vi "Stoerungen (257-320) - Amium.vi"(8 "Fehler (Eingang)":errorcluster caption="Fehler (Eingang, kein Fehler)") -> (0 "Fehler (Ausgang)":errorcluster, 3 "Störungen 257-320":u64)   [LabVIEW 2020, in "Stoerungen.lvlib"]
uses:
  Stoerungen.lvlib
  Seiten/System Einstellungen V2/Aktioen FGV System.ctl
  cRIO/Stoermeldungen/Stoerungen 257-320.ctl
  Stoerungen Messgeraet/Aktionen Kommunikation Stoerung.ctl
  Amium PNS/Aktion FGV Amium Daten.ctl
  PNS/Parameternamen PNS.ctl
  PNS/PNS.lvlib
  Seiten/System Einstellungen V2/System Einstellungen V2.lvlib
  cRIO/Stoermeldungen/Stoermeldungen.lvlib
  Amium PNS/Amium PNS.lvlib
panel:
  # "Störmeldungen PNS (257-320)"
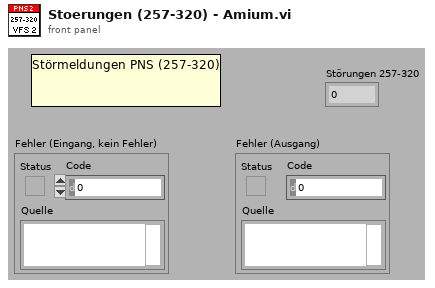
[diagram p1: front panel]
types:
  T1 = typedef "System Einstellungen V2.lvlib/Aktioen FGV System.ctl" = enum16{"lesen", "laden", "speichern", "Optionen schreiben", "Zeitstempel", "Reset BMP", "Reset SQP", "Wartung", "Werkseinstellung"}
  T2 = typedef "System Einstellungen V2.lvlib/Optionen.ctl" = cluster{"Störmeldep.":bool, "Betriebszustände":bool, "AK in ppm":bool, "log Cal-Gas":bool, "log 0-Gas":bool, "Durchflusssensor 0-5V":bool, "PNS?":bool, "Mit N2 spülen":bool, "TRE08":bool, "Amium 10-Fach":bool, "Verticale Scrollbar aktiv":bool, "Loggingtakt":bool, "AK Rezeptwechsel gleich wie MKS":bool, "NG ECO":bool}
  T3 = typedef "Amium PNS.lvlib/Aktion FGV Amium Daten.ctl" = enum16{"lesen", "Komm Daten", "Daten", "Error", "Regler", "Grenzwerte", "laden", "speichern"}
  T4 = typedef "Stoerungen.lvlib/Aktionen Kommunikation Stoerung.ctl" = enum16{"lesen", "init", "FT-IR Komm", "FT-IR Betriebsart", "FT-IR Hintergrund", "cRIO Komm", "PNS Komm", "Dichtheitstest", "Life Bit", "FTIR Komm AK", "PMA Komm", "FID Komm", "PMA Cal", "FID Ch4 Cal", "FID THC Cal", "Cal Timeout", "VFS 1 Komm", "VFS 2 Komm", "VFS 3 Komm", "VFS 4 Komm", "TRE 08 Komm", "CG-Test vorzeitig", "CG-Test Span 1", "CG-Test Span 2", "CG-Test Span 3", "CG-Test Messgas", "CG-Test löschen", "Test", "Amium AK", "AK Recept konfig", "AK Name konfig", "AK EKFG konfig"}
  T5 = typedef "Stoermeldungen.lvlib/Stoerungen 257-320.ctl" = cluster{"ERR. 257":bool, "ERR. 258":bool, "ERR. 259":bool, "ERR. 260":bool, "ERR. 261":bool, "ERR. 262":bool, "ERR. 263":bool, "ERR. 264":bool, "ERR. 265":bool, "ERR. 266":bool, "ERR. 267":bool, "ERR. 268":bool, "ERR. 269":bool, "ERR. 270":bool, "ERR. 271":bool, "ERR. 272":bool, "ERR. 273":bool, "ERR. 274":bool, "ERR. 275":bool, "ERR. 276":bool, "ERR. 277":bool, "ERR. 278":bool, "ERR. 279":bool, "ERR. 280":bool, "ERR. 281":bool, "ERR. 282":bool, "ERR. 283":bool, "ERR. 284":bool, "ERR. 285":bool, "ERR. 286":bool, "ERR. 287":bool, "ERR. 288":bool, "ERR. 289":bool, "ERR. 290":bool, "ERR. 291":bool, "ERR. 292":bool, "ERR. 293":bool, "ERR. 294":bool, "ERR. 295":bool, "ERR. 296":bool, "ERR. 297":bool, "ERR. 298":bool, "ERR. 299":bool, "ERR. 300":bool, "ERR. 301":bool, "ERR. 302":bool, "ERR. 303":bool, "ERR. 304":bool, "ERR. 305":bool, "ERR. 306":bool, "ERR. 307":bool, "ERR. 308":bool, "ERR. 309":bool, "ERR. 310":bool, "ERR. 311":bool, "ERR. 312":bool, "ERR. 313":bool, "ERR. 314":bool, "ERR. 315":bool, "ERR. 316":bool, "ERR. 317":bool, "ERR. 318":bool, "ERR. 319":bool, "ERR. 320":bool}
  T6 = typedef "PNS.lvlib/Parameternamen PNS.ctl" = enum16{"Heizkreis 1", "Heizkreis 2", "Heizkreis 3", "Heizkreis 4", "Heizkreis 5", "Heizkreis 6", "Heizkreis 7", "Heizkreis 8"}
  T7 = typedef "Amium PNS.lvlib/Amium ErrorCluster.ctl" = cluster{"Messgasdruck":bool, "Temperatur":bool, "Steuerluft":bool, "Temperatur HL 1":bool, "Temperatur HL 2":bool, "Temperatur HL 3":bool, "Temperatur HL 4":bool, "Temperatur HL 5":bool, "Temperatur HL 6":bool, "Temperatur HL 7":bool, "Temperatur HL 8":bool, "Temperatur HL 9":bool, "Temperatur HL 10":bool, "Temperatur 11 Ofen MGF/Filter":bool, "Temperatur HL12":bool, "Temperatur 13 Ofen MGP/Pumpe":bool, "Temperatur HL 14":bool}
  T8 = typedef "Amium PNS.lvlib/Temperaturregler Cluster.ctl" = cluster{"Istwert":sgl, "Sollwert":sgl, "Stellgröße":sgl, "Status":sgl, "Error":sgl}
  T9 = typedef "Stoerungen.lvlib/Stoerungen Messgeraete.ctl" = cluster{"FT-IR Komm":bool, "FT-IR Betriebsart":bool, "FT-IR Hintergrundscan":bool, "Dichtheitstest":bool, "cRIO Komm":bool, "PNS Komm":bool, "Life Bit":bool, "FT-IR AK Komm":bool, "PMA Komm":bool, "FID Komm":bool, "PMA Cal":bool, "FID CH4 Cal":bool, "FID THC Cal":bool, "Cal Timeout":bool, "VFS 1 Komm":bool, "VFS 2 Komm":bool, "VFS 3 Komm":bool, "VFS 4 Komm":bool, "TRE 08 Komm":bool, "CG-Test":bool, "CG-Test 1":bool, "CG-Test 2":bool, "CG-Test 3":bool, "Messgas - Eingang":bool, "Amium AK Komm":bool, "AK Rezept nicht konfiguriert ":bool, "AK Name nicht konfiguriert":bool, "AK EKFG nicht konfiguriert":bool}
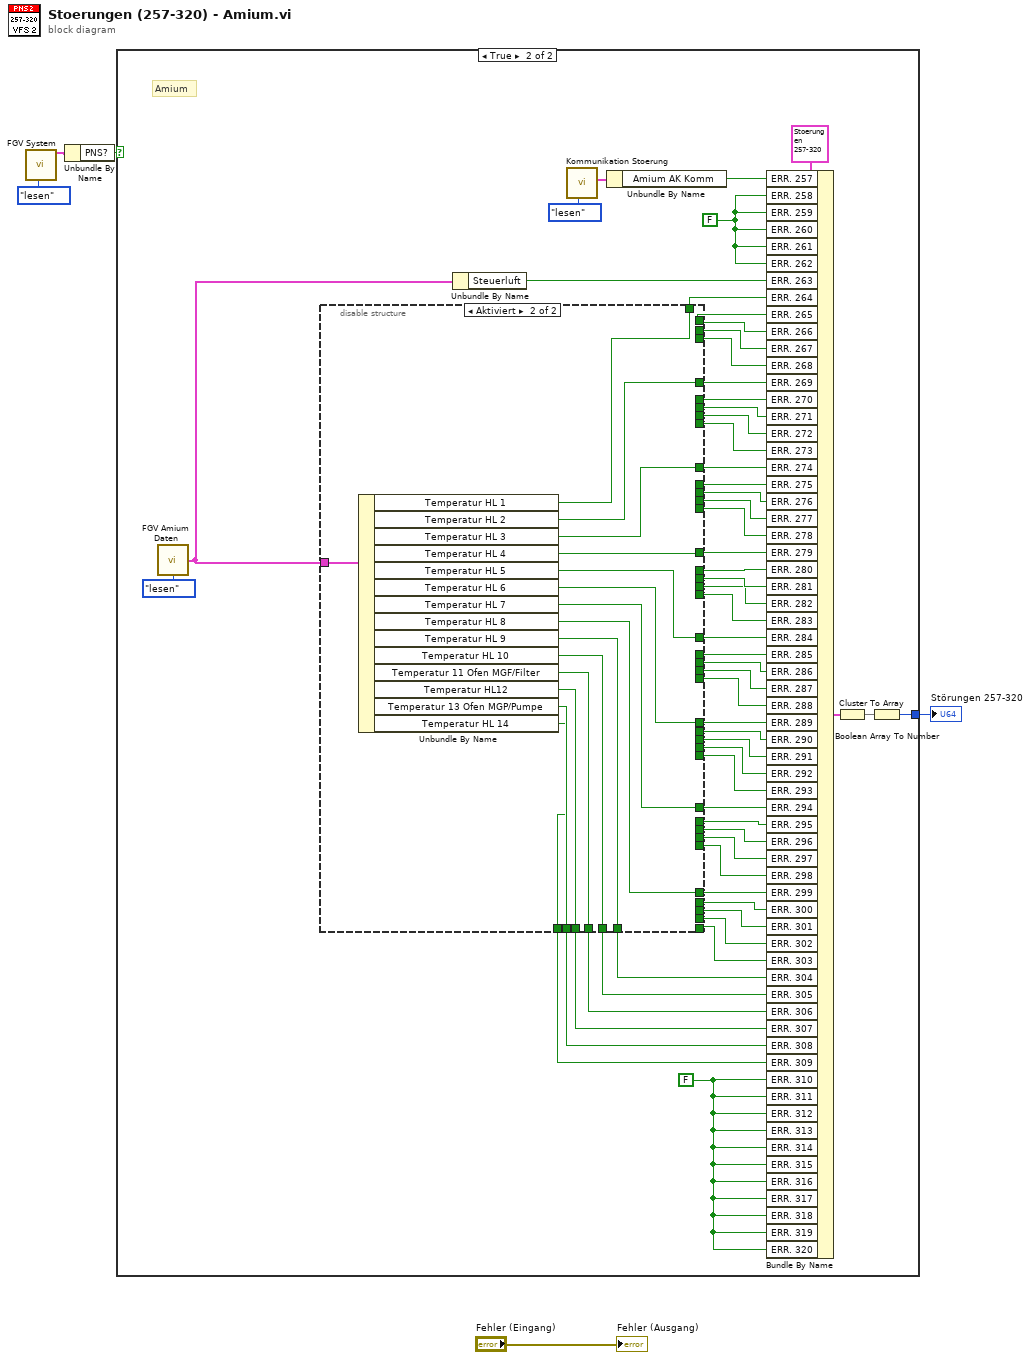
[diagram p0: block diagram]
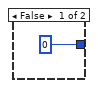
[diagram p2: hidden frame]
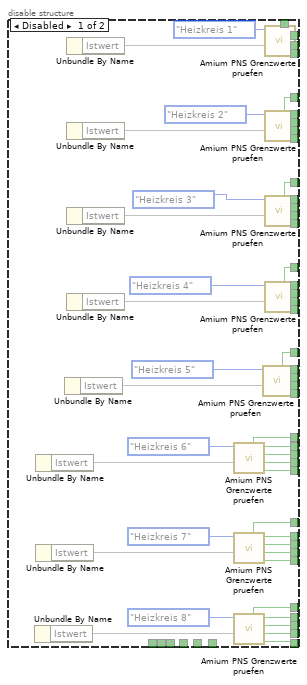
[diagram p3: hidden frame]
diagram:
  n1 = call "FGV System.vi"("Aktionen"=Aktioen_FGV_System."lesen") -> ("Optionen"=w3:T2)  [unwired: 12 in, 6 out]
  n2 = Unbundle By Name(w3) -> ("PNS?"=w1:bool)
  n3 = case shown="True" w1 {
    tunnel: [u64 0 w37] -> w4
    frame False {
    }
    frame True {
      w13 = FALSE ("ERR. 194")
      w38 = FALSE ("ERR. 194")
      # "Amium"
      n4 = call "FGV Amium Daten.vi"("Aktion"=Aktion_FGV_Amium_Daten."lesen") -> ("Fehler Cluster"=w14:T7)  [unwired: 9 in, 5 out]
      n5 = disable-structure shown="Aktiviert" {
        disable-tunnel: [w121 w142] -> w61
        disable-tunnel: [w120 _] -> w60
        disable-tunnel: [w119 _] -> w59
        disable-tunnel: [w118 _] -> w58
        disable-tunnel: [w117 _] -> w57
        disable-tunnel: [w116 w141] -> w56
        disable-tunnel: [w115 _] -> w55
        disable-tunnel: [w114 _] -> w54
        disable-tunnel: [w113 _] -> w53
        disable-tunnel: [w112 _] -> w52
        disable-tunnel: [w111 w140] -> w51
        disable-tunnel: [w110 _] -> w50
        disable-tunnel: [w109 _] -> w49
        disable-tunnel: [w108 _] -> w48
        disable-tunnel: [w107 _] -> w47
        disable-tunnel: [w106 w139] -> w46
        disable-tunnel: [w105 _] -> w45
        disable-tunnel: [w104 _] -> w44
        disable-tunnel: [w103 _] -> w43
        disable-tunnel: [w102 _] -> w42
        disable-tunnel: [w95 w138] -> w36
        disable-tunnel: [w94 _] -> w35
        disable-tunnel: [w93 _] -> w34
        disable-tunnel: [w92 _] -> w33
        disable-tunnel: [w91 _] -> w32
        disable-tunnel: [w87 w137] -> w31
        disable-tunnel: [w86 _] -> w30
        disable-tunnel: [w85 _] -> w29
        disable-tunnel: [w84 _] -> w28
        disable-tunnel: [w83 _] -> w27
        disable-tunnel: [w82 w136] -> w26
        disable-tunnel: [w81 _] -> w25
        disable-tunnel: [w80 _] -> w24
        disable-tunnel: [w79 _] -> w23
        disable-tunnel: [w78 _] -> w22
        disable-tunnel: [w77 w135] -> w21
        disable-tunnel: [w76 _] -> w20
        disable-tunnel: [w75 _] -> w19
        disable-tunnel: [w74 _] -> w18
        disable-tunnel: [w73 _] -> w17
        disable-tunnel: w14 -> [_ w143]
        disable-tunnel: [_ w134] -> w12
        disable-tunnel: [_ w133] -> w11
        disable-tunnel: [_ w132] -> w10
        disable-tunnel: [_ w131] -> w9
        disable-tunnel: [_ w130] -> w8
        disable-tunnel: [_ w129] -> w7
        frame Disabled {
          n6 = Unbundle By Name() -> (w88:T8, "Istwert"=w68)
          n7 = Unbundle By Name() -> (w90:T8, "Istwert"=w69)
          n8 = Unbundle By Name() -> (w89:T8, "Istwert"=w70)
          n9 = Unbundle By Name() -> (w96:T8, "Istwert"=w66)
          n10 = Unbundle By Name() -> (w128:T8, "Istwert"=w127)
          n11 = Unbundle By Name() -> (w126:T8, "Istwert"=w99)
          n12 = Unbundle By Name() -> (w125:T8, "Istwert"=w123)
          n13 = Unbundle By Name() -> (w124:T8, "Istwert"=w122)
          n14 = call "Amium PNS Grenzwerte pruefen.vi"("Wert"=w69, "Parameternamen PNS"=Parameternamen_PNS."Heizkreis 6") -> ("AbschMax"=w83:bool, "AbschMin"=w84:bool, "WarnMax"=w85:bool, "WarnMin"=w86:bool, "F.Br."=w87:bool)  [unwired: 5 in]
          n15 = call "Amium PNS Grenzwerte pruefen.vi"("Wert"=w70, "Parameternamen PNS"=Parameternamen_PNS."Heizkreis 7") -> ("AbschMax"=w78:bool, "AbschMin"=w79:bool, "WarnMax"=w80:bool, "WarnMin"=w81:bool, "F.Br."=w82:bool)  [unwired: 5 in]
          n16 = call "Amium PNS Grenzwerte pruefen.vi"("Wert"=w68, "Parameternamen PNS"=Parameternamen_PNS."Heizkreis 8") -> ("AbschMax"=w73:bool, "AbschMin"=w74:bool, "WarnMax"=w75:bool, "WarnMin"=w76:bool, "F.Br."=w77:bool)  [unwired: 5 in]
          n17 = call "Amium PNS Grenzwerte pruefen.vi"("Wert"=w66, "Parameternamen PNS"=Parameternamen_PNS."Heizkreis 5") -> ("AbschMax"=w91:bool, "AbschMin"=w92:bool, "WarnMax"=w93:bool, "WarnMin"=w94:bool, "F.Br."=w95:bool)  [unwired: 5 in]
          n18 = call "Amium PNS Grenzwerte pruefen.vi"("Wert"=w127, "Parameternamen PNS"=Parameternamen_PNS."Heizkreis 1") -> ("AbschMax"=w117:bool, "AbschMin"=w118:bool, "WarnMax"=w119:bool, "WarnMin"=w120:bool, "F.Br."=w121:bool)  [unwired: 5 in]
          n19 = call "Amium PNS Grenzwerte pruefen.vi"("Wert"=w99, "Parameternamen PNS"=Parameternamen_PNS."Heizkreis 2") -> ("AbschMax"=w112:bool, "AbschMin"=w113:bool, "WarnMax"=w114:bool, "WarnMin"=w115:bool, "F.Br."=w116:bool)  [unwired: 5 in]
          n20 = call "Amium PNS Grenzwerte pruefen.vi"("Wert"=w123, "Parameternamen PNS"=Parameternamen_PNS."Heizkreis 3") -> ("AbschMax"=w107:bool, "AbschMin"=w108:bool, "WarnMax"=w109:bool, "WarnMin"=w110:bool, "F.Br."=w111:bool)  [unwired: 5 in]
          n21 = call "Amium PNS Grenzwerte pruefen.vi"("Wert"=w122, "Parameternamen PNS"=Parameternamen_PNS."Heizkreis 4") -> ("AbschMax"=w102:bool, "AbschMin"=w103:bool, "WarnMax"=w104:bool, "WarnMin"=w105:bool, "F.Br."=w106:bool)  [unwired: 5 in]
        }
        frame Enabled {
          n22 = Unbundle By Name(w143) -> ("Temperatur HL 1"=w142:bool, "Temperatur HL 2"=w141:bool, "Temperatur HL 3"=w140:bool, "Temperatur HL 4"=w139:bool, "Temperatur HL 5"=w138:bool, "Temperatur HL 6"=w137:bool, "Temperatur HL 7"=w136:bool, "Temperatur HL 8"=w135:bool, "Temperatur HL 9"=w134:bool, "Temperatur HL 10"=w133:bool, "Temperatur 11 Ofen MGF/Filter"=w132:bool, "Temperatur HL12"=w131:bool, "Temperatur 13 Ofen MGP/Pumpe"=w130:bool, "Temperatur HL 14"=w129:bool)
        }
      }
      n23 = Unbundle By Name(w14) -> ("Steuerluft"=w15:bool)
      n24 = call "Kommunikation Stoerung.vi"("Aktionen"=Aktionen_Kommunikation_Stoerung."lesen") -> ("Störung Messgerät"=w41:T9)  [unwired: 10 in]
      n25 = Unbundle By Name(w41) -> ("Amium AK Komm"=w39:bool)
      n26 = Bundle By Name(cluster=T5 {"ERR. 257"=FALSE, "ERR. 258"=FALSE, "ERR. 259"=FALSE, "ERR. 260"=FALSE, "ERR. 261"=FALSE, "ERR. 262"=FALSE, "ERR. 263"=FALSE, "ERR. 264"=FALSE, "ERR. 265"=FALSE, "ERR. 266"=FALSE, "ERR. 267"=FALSE, "ERR. 268"=FALSE, "ERR. 269"=FALSE, "ERR. 270"=FALSE, "ERR. 271"=FALSE, "ERR. 272"=FALSE, "ERR. 273"=FALSE, "ERR. 274"=FALSE, "ERR. 275"=FALSE, "ERR. 276"=FALSE, "ERR. 277"=FALSE, "ERR. 278"=FALSE, "ERR. 279"=FALSE, "ERR. 280"=FALSE, "ERR. 281"=FALSE, "ERR. 282"=FALSE, "ERR. 283"=FALSE, "ERR. 284"=FALSE, "ERR. 285"=FALSE, "ERR. 286"=FALSE, "ERR. 287"=FALSE, "ERR. 288"=FALSE, "ERR. 289"=FALSE, "ERR. 290"=FALSE, "ERR. 291"=FALSE, "ERR. 292"=FALSE, "ERR. 293"=FALSE, "ERR. 294"=FALSE, "ERR. 295"=FALSE, "ERR. 296"=FALSE, "ERR. 297"=FALSE, "ERR. 298"=FALSE, "ERR. 299"=FALSE, "ERR. 300"=FALSE, "ERR. 301"=FALSE, "ERR. 302"=FALSE, "ERR. 303"=FALSE, "ERR. 304"=FALSE, "ERR. 305"=FALSE, "ERR. 306"=FALSE, "ERR. 307"=FALSE, "ERR. 308"=FALSE, "ERR. 309"=FALSE, "ERR. 310"=FALSE, "ERR. 311"=FALSE, "ERR. 312"=FALSE, "ERR. 313"=FALSE, "ERR. 314"=FALSE, "ERR. 315"=FALSE, "ERR. 316"=FALSE, "ERR. 317"=FALSE, "ERR. 318"=FALSE, "ERR. 319"=FALSE, "ERR. 320"=FALSE} ("STÖRUNGEN 193-256"), "ERR. 257"=w39, "ERR. 258"=w38, "ERR. 259"=w38, "ERR. 260"=w38, "ERR. 261"=w38, "ERR. 262"=w38, "ERR. 263"=w15, "ERR. 264"=w61, "ERR. 265"=w60, "ERR. 266"=w59, "ERR. 267"=w58, "ERR. 268"=w57, "ERR. 269"=w56, "ERR. 270"=w55, "ERR. 271"=w54, "ERR. 272"=w53, "ERR. 273"=w52, "ERR. 274"=w51, "ERR. 275"=w50, "ERR. 276"=w49, "ERR. 277"=w48, "ERR. 278"=w47, "ERR. 279"=w46, "ERR. 280"=w45, "ERR. 281"=w44, "ERR. 282"=w43, "ERR. 283"=w42, "ERR. 284"=w36, "ERR. 285"=w35, "ERR. 286"=w34, "ERR. 287"=w33, "ERR. 288"=w32, "ERR. 289"=w31, "ERR. 290"=w30, "ERR. 291"=w29, "ERR. 292"=w28, "ERR. 293"=w27, "ERR. 294"=w26, "ERR. 295"=w25, "ERR. 296"=w24, "ERR. 297"=w23, "ERR. 298"=w22, "ERR. 299"=w21, "ERR. 300"=w20, "ERR. 301"=w19, "ERR. 302"=w18, "ERR. 303"=w17, "ERR. 304"=w12, "ERR. 305"=w11, "ERR. 306"=w10, "ERR. 307"=w9, "ERR. 308"=w8, "ERR. 309"=w7, "ERR. 310"=w13, "ERR. 311"=w13, "ERR. 312"=w13, "ERR. 313"=w13, "ERR. 314"=w13, "ERR. 315"=w13, "ERR. 316"=w13, "ERR. 317"=w13, "ERR. 318"=w13, "ERR. 319"=w13, "ERR. 320"=w13) -> (w64:T5)
      n27 = Cluster To Array(cluster=w64) -> (array=w63:bool[])
      n28 = Boolean Array To Number ("Boolesches Array nach Zahl")(Boolean array=w63) -> (number=w37:u64)
    }
  }
  "Störungen 257-320" <- w4
  "Fehler (Ausgang)" <- "Fehler (Eingang)"
